vi "Configure ExtOut Connector.vi"(8 "error in (no error)":errorcluster, 9 "Polarity (0:Negative)":u16(ring) items=["Negative", "Positive"], 10 "Trigger Type (2:Input Complete)":u16(ring)=2 items=["Aperture Waveform", "Burst Complete", "Input Complete", "Off", "Once", "Reading Complete", "Service Request"], 11 "VISA resource name":refnum<visa-resource-name>) -> (0 "error out":errorcluster, 3 "VISA resource name out":refnum<visa-resource-name>)   [LabVIEW 2020, in "3458A Virtual Digitizer.lvlib" / "3458A Basic Driver.lvlib"]
doc: "Configures the kind of input signal that will be detected from the Ext Out connector. This signal can then be used to trigger measurements."
uses:
  3458A Basic Driver.lvlib
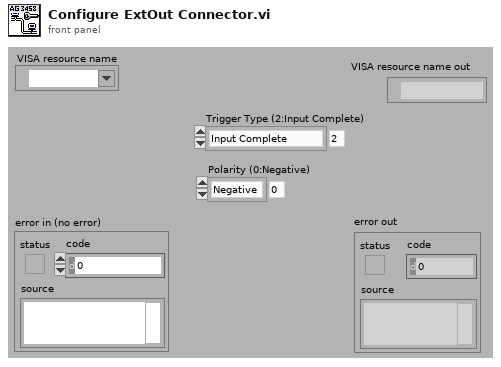
[diagram p1: front panel]
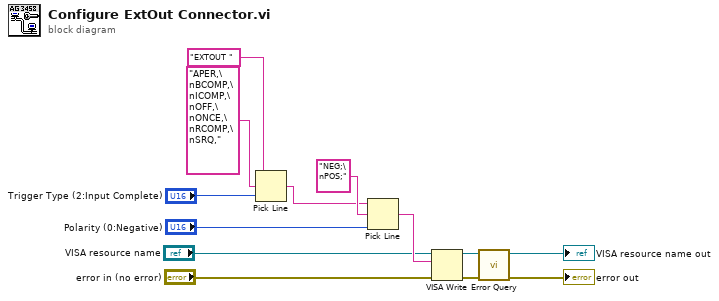
[diagram p0: block diagram]
diagram:
  n1 = Pick Line(string ("")="EXTOUT ", multi-line string="APER,\nBCOMP,\nICOMP,\nOFF,\nONCE,\nRCOMP,\nSRQ,", line index="Trigger Type (2:Input Complete)") -> (output string=w10:string)
  n2 = Pick Line(string ("")=w10, multi-line string="NEG;\nPOS;", line index="Polarity (0:Negative)") -> (output string=w7:string)
  n3 = VISA Write(VISA resource name="VISA resource name", write buffer=w7, error in (no error)="error in (no error)") -> (VISA resource name out=w9:refnum<visa-resource-name>, error out=w8:errorcluster)  [unwired: 1 out]
  n4 = call "Error Query.vi"("error in (no error)"=w8, "VISA resource name"=w9) -> ("error out"=→"error out":errorcluster, "VISA resource name out"=→"VISA resource name out":refnum<visa-resource-name>)  [unwired: 6 in, 2 out]
